vi "Read.vi"(8 "error in (no error)":errorcluster, 11 "Inc Var Command Config in":refnum<class "Dec Var Command Config.lvclass">) -> (0 "error out":errorcluster, 2 "Name":string, 3 "Inc Var Command Config out":refnum<class "Dec Var Command Config.lvclass">)   [LabVIEW 2020, in "VolatusSeqConfig.lvlib" / "Dec Var Command Config.lvclass"]
uses:
  Dec Var Command Config.lvclass
  Dec Var Command Config.lvclass/Dec Var Command Config.ctl
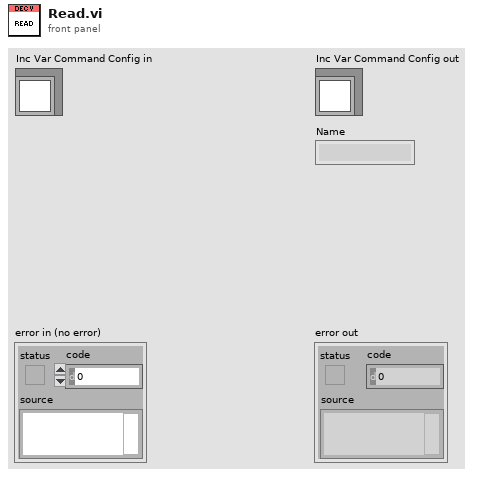
[diagram p1: front panel]
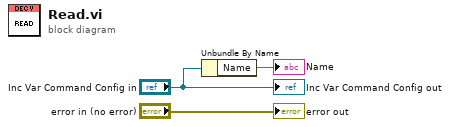
[diagram p0: block diagram]
diagram:
  n1 = Unbundle By Name("Inc Var Command Config in") -> ("Name"=→"Name":string)
  "error out" <- "error in (no error)"
  "Inc Var Command Config out" <- "Inc Var Command Config in"
